vi "ToggleSupplyOnOff.vi"(9 "State":enum8{"OFF", "ON"}(ring), 11 "Port":enum8{"ONE", "TWO"}(ring)) -> (3 "ByteArrayToSend":u8[](array[numeric]) format="%x")   [LabVIEW 2019]
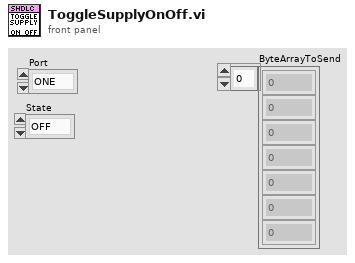
[diagram p1: front panel]
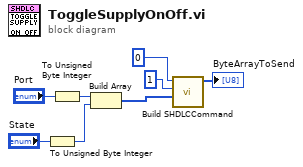
[diagram p0: block diagram]
diagram:
  n1 = To Unsigned Byte Integer(number="State") -> (unsigned 8bit integer=w1:u8)
  n2 = To Unsigned Byte Integer(number="Port") -> (unsigned 8bit integer=w5:u8)
  n3 = Build Array(w5, w1) -> (w4:u8[])
  n4 = call "Build SHDLCCommand.vi"("Data"=w4, "CommandID"=u8 1, "SlaveAdress"=u8 0) -> ("ByteArrayToSend"=→"ByteArrayToSend":u8[])  [unwired: 8 in]
